vi "Auton Drive Gyro.vi"(4 "Left Gains":T1={"proportional gain (Kc)"=0.25, "integral time (Ti, min)"=0.0, "derivative time (Td, min)"=0.0} {"derivative time (Td, min)" format="%.3f"; "integral time (Ti, min)" format="%.3f"; "proportional gain (Kc)" format="%.3f"}, 5 "Right Gains":T1={"proportional gain (Kc)"=0.25, "integral time (Ti, min)"=0.0, "derivative time (Td, min)"=0.0} {"derivative time (Td, min)" format="%.3f"; "integral time (Ti, min)" format="%.3f"; "proportional gain (Kc)" format="%.3f"}, 6 "Left Range":cluster{"output high":dbl, "output low":dbl}={"output high"=0.55, "output low"=-0.55} {"output low" format="%.2f"; "output high" format="%.2f"}, 7 "Right Range":cluster{"output high":dbl, "output low":dbl}={"output high"=0.4, "output low"=-0.4} {"output low" format="%.2f"; "output high" format="%.2f"}, 8 "Angle Setpoint":dbl, 10 "Right Set Point":dbl=-200.0, 11 "Left Set Point":dbl=-200.0) -> (3 "At Destination?":bool=TRUE)   [LabVIEW 2014]
uses:
  <vilib>/Rock Robotics/WPI/RobotDrive/WPI_RobotDriveGetSetRefNum.vi
  <vilib>/addons/control/pid/pid.llb/PID (DBL).vi
  <vilib>/Rock Robotics/Network Tables/SD Write Number.vi
  <vilib>/Rock Robotics/WPI/RobotDrive/WPI_RobotDriveArcadeDrive_Standard(NoSaturation).vi
  <vilib>/addons/control/pid/NI_PID_pid.lvlib
panel:
  out "Gyro Reading":dbl(knob)=0.34322617224 scale=-180.0..180.0
  in  "Y Value Forward/Reverse":dbl=-0.7
  out "X Value Left/Right Correction":dbl=-0.08580654306 format="%.2f"
  in  "Encoder Destination Range":dbl=2.0
  in  "Gain (VoltsPerDegree/Second)":dbl=0.0066
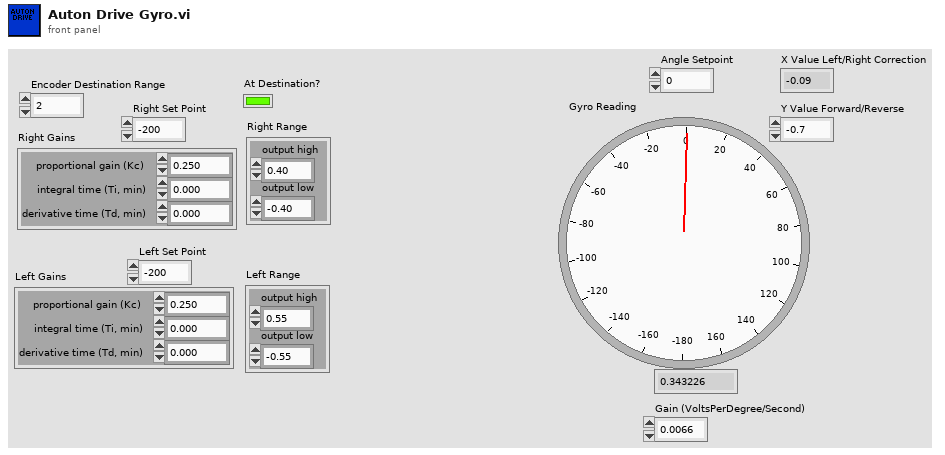
[diagram p1: front panel]
types:
  T1 = cluster{"proportional gain (Kc)":dbl, "integral time (Ti, min)":dbl, "derivative time (Td, min)":dbl}
  T2 = typedef "WPI_GyroDevRef.ctl" = cluster{"DevStatus":errorcluster, "Analog Module":T3, "Analog Channel":T4, "Offset":dbl, "Gain (VoltsPerDegree/Second)":dbl}
  T3 = typedef "FPGA_TypedefAnalogModule.ctl" = enum16{"Controller 1"}
  T4 = typedef "FPGA_AIChannel.ctl" = enum8{"AI 0", "AI 1", "AI 2", "AI 3", "AI MXP 0", "AI MXP 1", "AI MXP 2", "AI MXP 3", "Invalid"}
  T5 = typedef "WPI_EncoderDevRef.ctl" = cluster{"DevStatus":errorcluster, "EncoderIndex":T6, "CounterIndex":T7, "DistancePerCount":dbl, "Decoding Type":T8}
  T6 = typedef "FPGA_EncoderIdx.ctl" = enum8{"Enc 0", "Enc 1", "Enc 2", "Enc 3", "Enc 4", "Enc 5", "Enc 6", "Enc 7", "Invalid"}
  T7 = typedef "FPGA_CounterCtrSystemIndex.ctl" = enum8{"Ctr 0", "Ctr 1", "Ctr 2", "Ctr 3", "Ctr 4", "Ctr 5", "Ctr 6", "Ctr 7", "Invalid"}
  T8 = typedef "WPI_EncoderType.ctl" = enum16{"1x", "2x", "4x"}
  T9 = typedef "WPI_RobotDriveDevRef.ctl" = cluster{"DevStatus":errorcluster, "Motors[]":T10[], "Square Inputs":bool, "Max Output":dbl}
  T10 = typedef "WPI_MotorControlDeviceRef.ctl" = cluster{"DeviceStatus":errorcluster, "Type":T11, "PWM":cluster{"Controller":T12, "PWM Channel":T13, "DeadBand":T14}, "CAN":cluster{"Device Number":u8, "Control Mode":T15, "Semaphore":T16, "Max Vout":dbl, "TalonSRX Control Mode":T17}, "Invert":bool, "TransformRef":T18, "InvTransformRef":T18}
  T11 = typedef "WPI_MotorControlType.ctl" = enum16{"PWM", "CAN", "CANTalonSRX"}
  T12 = typedef "FPGA_TypedefDigitalModule.ctl" = enum16{"Controller 1"}
  T13 = typedef "FPGA_DIOPWMChannel.ctl" = enum8{"PWM 0", "PWM 1", "PWM 2", "PWM 3", "PWM 4", "PWM 5", "PWM 6", "PWM 7", "PWM 8", "PWM 9", "PWM MXP 0", "PWM MXP 1", "PWM MXP 2", "PWM MXP 3", "PWM MXP 4", "PWM MXP 5", "PWM MXP 6", "PWM MXP 7", "PWM MXP 8", "PWM MXP 9", "Invalid"}
  T14 = typedef "WPI_PWMDeadband.ctl" = cluster{"Name":string, "maxPositivePwm":i32, "minPositivePwm":i32, "centerPwm":i32, "maxNegativePwm":i32, "minNegativePwm":i32, "angularRange":u16}
  T15 = typedef "WPI_CANJaguar_ControlMode.ctl" = enum8{"Percent VBus", "Current", "Speed", "Position", "Voltage"}
  T16 = typedef "Semaphore RefNum" = refnum<k1>
  T17 = typedef "WPI_CANTalonSRX_APIControlMode.ctl" = enum8{"Percent VBus", "Speed", "Position", "Slave", "Unchanged / Invalid"}
  T18 = typedef "WPI_PWMTransform_ConPane.ctl" = refnum<vi>
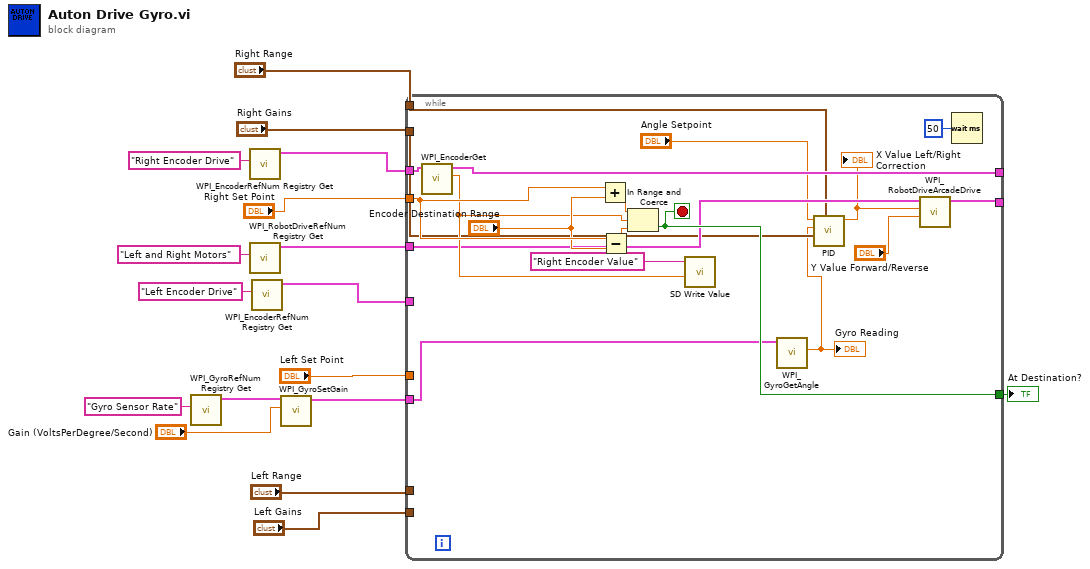
[diagram p0: block diagram]
diagram:
  n1 = call <vilib>:"WPI_GyroRefNum Registry Get.vi"("refnum name"="Gyro Sensor Rate") -> ("GyroDevRef"=w4:T2)  [unwired: 9 in, 1 out]
  n2 = call <vilib>:"WPI_EncoderRefNum Registry Get.vi"("refnum name"="Right Encoder Drive") -> ("EncoderDevRef"=w10:T5)  [unwired: 9 in, 1 out]
  n3 = call <vilib>:"WPI_RobotDriveRefNum Registry Get.vi"("refnum name"="Left and Right Motors") -> ("RobotDriveDevRef"=w14:T9)  [unwired: 9 in, 1 out]
  n4 = call <vilib>:"WPI_EncoderRefNum Registry Get.vi"("refnum name"="Left Encoder Drive") -> ("EncoderDevRef"=w11:T5)  [unwired: 9 in, 1 out]
  n5 = call <vilib>:"WPI_GyroSetGain.vi"("Gain (VoltsPerDegree/Second)"="Gain (VoltsPerDegree/Second)", "GyroDevRef"=w4) -> ("GyroDevRef"=w3:T2)  [unwired: 1 in, 8 out]
  n6 = while {
    tunnel: [w35] -> _
    tunnel: [w25] -> _
    tunnel: "Left Gains" -> [_]
    tunnel: "Left Range" -> [_]
    tunnel: w14 -> [w24]
    tunnel: w11 -> [_]
    tunnel: w10 -> [w34]
    tunnel: "Left Set Point" -> [_]
    tunnel: "Right Set Point" -> [w32]
    tunnel: [w29] -> w7
    tunnel: w3 -> [w28]
    tunnel: "Right Range" -> [w21]
    tunnel: "Right Gains" -> [w22]
    stop <- w29 stop-if-true
    n7 = call <vilib>:"WPI_EncoderGet.vi"("EncoderDevRef"=w34) -> ("Distance"=w26:dbl, "EncoderDevRef"=w35:T5)  [unwired: 5 in, 4 out]
    n8 = Add(x=w32, y="Encoder Destination Range") -> (x+y=w33:dbl)
    n9 = Subtract(x=w32, y="Encoder Destination Range") -> (x-y=w31:dbl)
    n10 = In Range and Coerce(upper limit=w33, x=w26, lower limit=w31) -> (In Range?=w29:bool)  [unwired: 1 out]
    n11 = call-poly <vilib>:"SD Write Value.vi"("Numeric"=w26, "Name"="Right Encoder Value") -> ()  [unwired: 8 in, 2 out]
    n12 = call <vilib>:"WPI_GyroGetAngle.vi"("GyroDevRef"=w28) -> ("Angle"=w19:dbl)  [unwired: 1 in, 9 out]
    "Gyro Reading" <- w19
    n13 = call-poly <vilib>:"PID.vi"("output range"=w21, "PID gains"=w22, "process variable"=w19, "setpoint"="Angle Setpoint") -> ("output"=w23:dbl)  [unwired: 6 in, 1 out]
    "X Value Left/Right Correction" <- w23
    n14 = call-poly <vilib>:"WPI_RobotDriveArcadeDrive.vi"("Y axis value"="Y Value Forward/Reverse", "X axis value"=w23, "RobotDriveDevRef"=w24) -> ("RobotDriveDevRef"=w25:T9)  [unwired: 6 in, 2 out]
    n15 = Wait (ms)(milliseconds to wait=u32 50) -> ()  [unwired: 1 out]
  }
  "At Destination?" <- w7
